vi "Actor Core.vi"(8 "error in":errorcluster, 11 "Server in":refnum<class "Server.lvclass">) -> (0 "error out":errorcluster, 3 "Actor out":refnum<class "Actor.lvclass">)   [LabVIEW 2016, in "Server.lvlib" / "Server.lvclass"]
doc: "(<B>Filename</B>: Actor Framework.lvlib:Actor.lvclass:Actor Core.vi)\n\nReceives messages to the actor, reacts to them, and initiates any error handling that may shut the actor down.\n\nDescendant classes may override this VI to append parallel tasks for the actor to complete while it handles messages. Overrides use the Call Parent Method node."
uses:
  Server.lvclass
  <vilib>/ActorFramework/Actor/Actor.lvclass
  Server.lvclass/Server.ctl
  <vilib>/NI/STM/TCP/Read Meta Data (TCP Ref).vi
  <vilib>/NI/STM/TCP/Get Connection Reference (TCP).vi
  <vilib>/NI/STM/TCP/Read Meta Data (TCP Clst).vi
  <vilib>/NI/STM/TCP/Read Message (TCP).vi
  <vilib>/NI/STM/NI STM.lvlib
panel:
  in  "Target IP Address":string="localhost"
  in  "stop":bool
  out "Data":dbl[](array[numeric])
  out "Port Number":u16
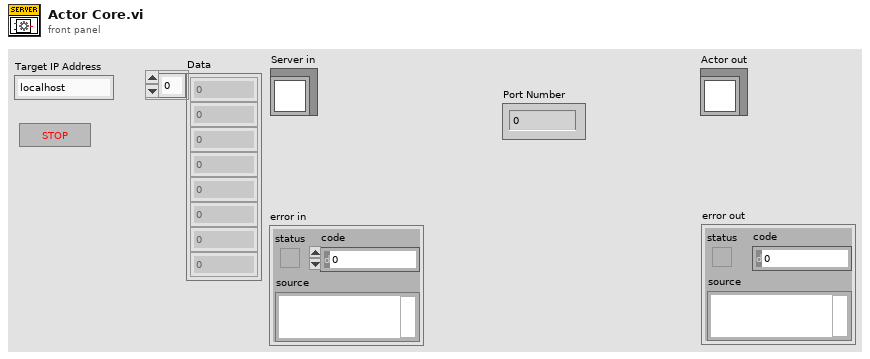
[diagram p1: front panel]
types:
  T1 = typedef "NI STM.lvlib/TCP Connection Info.ctl" = cluster{"connection ID":refnum<k5>, "meta data":T2[]}
  T2 = typedef "NI STM.lvlib/MetaDataElement.ctl" = string
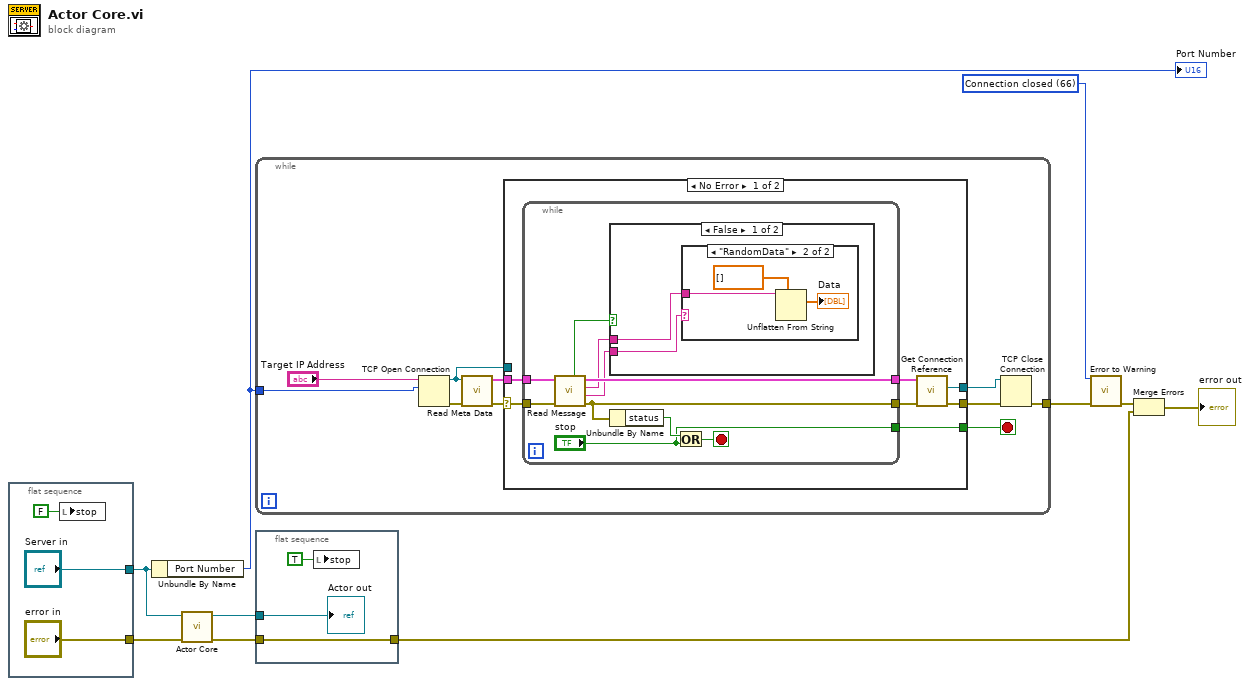
[diagram p0: block diagram]
diagram:
  w1 = 66 items=["No Error", "Argument Error", "Memory Full", "Out of Zone", "End of File", "File Already Open", "Generic File IO Error", "File Not Found", "File Permission Error", "Disk Full", "Duplicate Path", "Too Many Files Open", "Not Enabled", "Resource File Not Found", "Cannot Add Resource", "Resource Not Found", "Image Not Found", "Image Memory Error", "Pen Does Not Exist", "Config Bad Type", "Config Token Not Found", "Config Parse Error", "Config Memory Error", "Bad External Code Format", "Bad External Code Offset", "External Code Not Present", "Null Window", "Destroy Window Mixup", "Null Menu", "Print Aborted", "Bad Print Record", "Print Driver Error", "Windows Error During Print", "Memory Error During Print", "Print Dialog Error", "Generic Print Error", "Invalid Device Refnum", "Device Not Found", "Device Parameter Error", "Device Unit Error", "Can't Open Device", "Device Call Aborted", "Generic Error", "Cancelled By User", "Object ID Too Low", "Object ID Too High", "Object Not In Heap", "Unknown Heap", "Bad DefProc ID", "DefProc Not In Table", "Message Out Of Range", "Null Method", "Unknown Message", "Manager Call Not Supported", "Bad address", "Connection In progress", "Connection timed out", "Connection is already in progress", "Network attribute not supported", "Network error", "Address in use", "System out of memory", "Connection aborted", "Connection refused", "Connection is not connected", "Connection is already connected", "Connection closed", "Initialize error (interapplication manager)", "Bad occurrence", "Wait on unbound occurrence handler", "Occurrence queue overflow", "Bad path", "Semaphore not signaled", "Unrecognized type (interapplication manager)"] ("1st Error to Convert")
  n1 = flat-sequence {
    tunnel: ["error in"] -> w9
    tunnel: ["Server in"] -> w8
    frame #0 {
      n2 = local write "stop"(FALSE ("stop")) -> ()
    }
  }
  n3 = Unbundle By Name(w8) -> ("Port Number"=w6:u16)
  "Port Number" <- w6
  n4 = call-parent "Actor Core.vi"("error in"=w9, "Actor in"=w8) -> ("error out"=w3:errorcluster, "Actor out"=w10:refnum<class "Actor.lvclass">)  [unwired: 8 in]
  n5 = while {
    tunnel: [w19] -> w7
    tunnel: w6 -> [w22]
    stop <- w21 stop-if-true
    n6 = TCP Open Connection(address="Target IP Address", remote port or service name=w22) -> (connection ID=w14:refnum<k5>, error out=w18:errorcluster)  [unwired: 1 in, 2 out]
    n7 = call-poly <vilib>:"Read Meta Data.vi"("error in"=w18, "connection ID"=w14) -> ("error out"=w17:errorcluster, "connection info out"=w16:T1)  [unwired: 1 in, 7 out]
    n8 = case shown="No Error" w17 {
      selector: w17 -> [w26 _]
      tunnel: [w28 _] -> w21
      tunnel: [w27 _] -> w20
      tunnel: w16 -> [w25 _]
      tunnel: [w24 w46] -> w15
      tunnel: w14 -> [_ w46]
      frame No Error {
        n9 = while {
          tunnel: w25 -> [w40]
          tunnel: w26 -> [w39]
          tunnel: [w38] -> w30
          tunnel: [w35] -> w29
          tunnel: ["stop"] -> w28
          stop <- w33 stop-if-true
          n10 = call-poly <vilib>:"Read Message.vi"("error in"=w39, "connection info in"=w40) -> ("error out"=w35:errorcluster, "name"=w37:T2, "data string"=w36:string, "connection info out"=w38:T1, "timed out?"=w32:bool)  [unwired: 1 in, 4 out]
          n11 = case shown="False" w32 {
            tunnel: w37 -> [w41 _]
            tunnel: w36 -> [w42 _]
            frame False {
              n12 = case shown="\"RandomData\"" w41 {
                tunnel: w42 -> [_ w45]
                frame Default {
                }
                frame "RandomData" {
                  n13 = Unflatten From String(type=dbl[] [], binary string=w45) -> (value=→"Data":dbl[])  [unwired: 1 in, 4 out]
                }
              }
            }
            frame True {
            }
          }
          n14 = Unbundle By Name(w35) -> ("status"=w34:bool)
          n15 = Or(x=w34, y="stop") -> (x .or. y?=w33:bool)
        }
        n16 = call-poly <vilib>:"Get Connection Reference.vi"("error in"=w29, "connection info in"=w30) -> ("error out"=w27:errorcluster, "connection ID out"=w24:refnum<k5>)  [unwired: 8 out]
      }
      frame Error {
      }
    }
    n17 = TCP Close Connection(connection ID=w15, error in (no error)=w20) -> (error out=w19:errorcluster)  [unwired: 2 out]
  }
  n18 = flat-sequence {
    tunnel: w10 -> [w49]
    tunnel: [w48] -> w4
    tunnel: w3 -> [w48]
    frame #0 {
      n19 = local write "stop"(TRUE ("stop")) -> ()
      "Actor out" <- w49
    }
  }
  n20 = call <vilib>:"Error to Warning.vi"("1st Error to Convert"=w1, "error in"=w7) -> ("warning out"=w2:errorcluster)  [unwired: 3 in, 10 out]
  n21 = Merge Errors(w2, w4) -> (→"error out":errorcluster)
